vi "Test Z Axis Motor.vi"(6 "Stop Button":bool, 9 "Motor Test Controls":T1, 10 "PWM Duty Cycle":dbl(knob) min=0.0 max=100.0 step=1.0 scale=0.0..100.0) -> ()   [LabVIEW 2013]
doc: "This VI tests the Z-axis functionality. The Z-axis communicates a bit differently than the X and Y axes, thus\nit is given its own test VI."
uses:
  Controls/PWM_test_ctrl_cluster.ctl
  Controls/PWM_data_cluster.ctl
  Controls/table_axis_enum.ctl
  Controls/PWM_state_enum.ctl
  <vilib>/DAQmx/write.llb/DAQmx Write (Digital Bool 1Line 1Point).vi
  <vilib>/DAQmx/miscellaneous.llb/DAQmx Fill In Error Info.vi
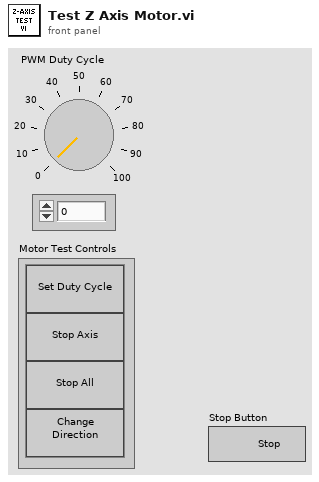
[diagram p1: front panel]
types:
  T1 = typedef "PWM_test_ctrl_cluster.ctl" = cluster{"Set Speed":bool, "Stop Axis":bool, "Stop All":bool, "Change Dir":bool}
  T2 = typedef "PWM_data_cluster.ctl" = cluster{"frequency":dbl, "Duty Cycle (%)":dbl, "Axis Enum":T3, "Function Enum":T4}
  T3 = typedef "table_axis_enum.ctl" = enum16{"X-axis", "Y-axis", "Z-axis", "W-axis"}
  T4 = typedef "PWM_state_enum.ctl" = enum16{"Initialize", "SetAxisSpeed", "StopAxis", "StopAll", "Shutdown"}
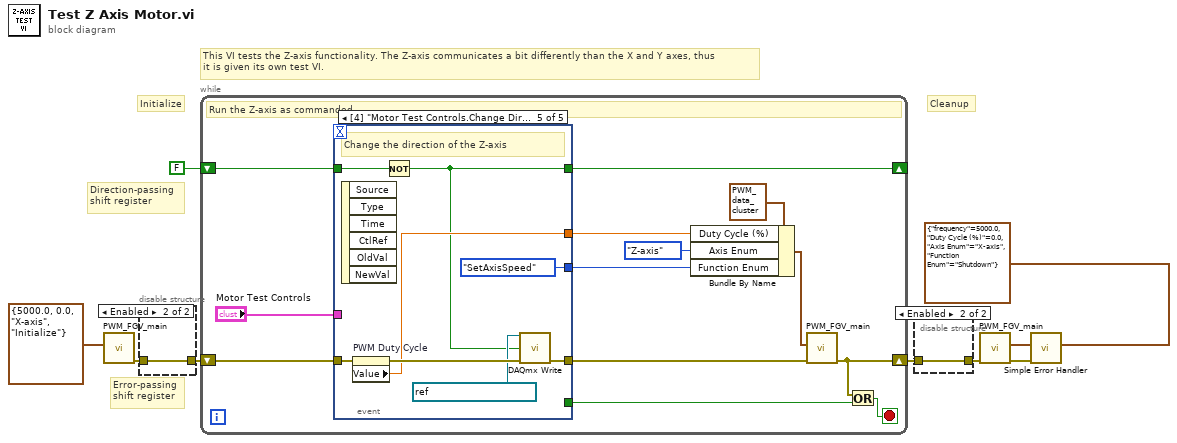
[diagram p0: block diagram]
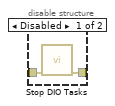
[diagram p2: hidden frame]
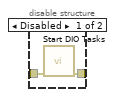
[diagram p3: hidden frame]
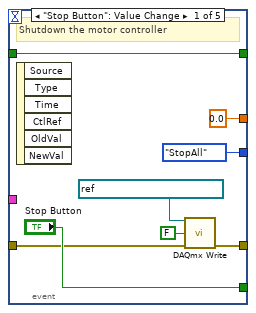
[diagram p4: hidden frame]
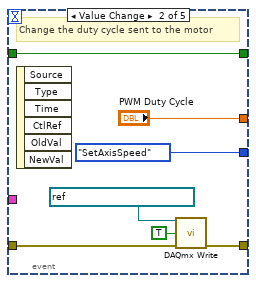
[diagram p5: hidden frame]
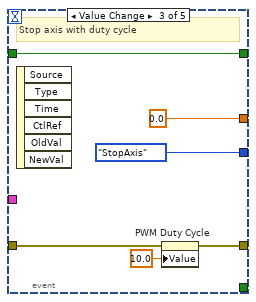
[diagram p6: hidden frame]
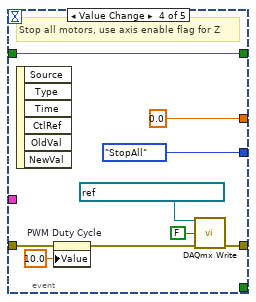
[diagram p7: hidden frame]
diagram:
  # "Direction-passing\nshift register"
  # "Cleanup"
  # "Initialize"
  # "Error-passing\nshift register"
  # "This VI tests the Z-axis functionality. The Z-axis communicates a bit differently than the X and Y axes, thus\nit is given its own test VI."
  n1 = call "PWM_FGV_main.vi"("PWM FGV Data"=T2 {"frequency"=5000.0, "Duty Cycle (%)"=0.0, "Axis Enum"=enum."X-axis", "Function Enum"=enum."Initialize"}) -> ("Error Out"=w7:errorcluster)  [unwired: 10 in]
  n2 = disable-structure shown="Enabled" {
    disable-tunnel: w7 -> [w10 w11]
    disable-tunnel: [w9 w11] -> w6
    frame Disabled {
      n3 = call "Start DIO Tasks.vi"("error in (no error)"=w10) -> ("error out"=w9:errorcluster)  [unwired: 10 in]
    }
    frame Enabled {
    }
  }
  n4 = while {
    shift-right: [w21] -> w5
    shift-left: w6 -> [w24]
    shift-right: [w12] -> _
    shift-left: FALSE -> [w13]
    stop <- w22 stop-if-true
    # "Run the Z-axis as commanded"
    n5 = event shown="[4] \"Motor Test Controls.Change Dir\": Value Change" {
      selector: _ -> [_ _ _ _ _]
      dyn-events: _ -> [_ _ _ _ _]
      timeout: _ -> [_ _ _ _ _]
      tunnel: w24 -> [w28 w36 w43 w52 w61]
      tunnel: "Motor Test Controls" -> [_ _ _ _ _]
      tunnel: [w29 w37 w42 w50 w62] -> w20
      tunnel: ["Stop Button" _ _ _ _] -> w19
      tunnel: [0.0 ("Duty Cycle (%)") "PWM Duty Cycle" 0.0 ("PWM Duty Cycle") 0.0 ("PWM Duty Cycle") w58] -> w16
      tunnel: [PWM_state_enum."StopAll" ("Function Enum") PWM_state_enum."SetAxisSpeed" ("Function Enum") PWM_state_enum."StopAxis" ("Function Enum") PWM_state_enum."StopAll" ("Function Enum") PWM_state_enum."SetAxisSpeed" ("Function Enum")] -> w15
      tunnel: w13 -> [w25 w33 w40 w46 w56]
      tunnel: [w25 w33 w40 w46 w55] -> w12
      event "Stop Button": Value Change {
        # "Shutdown the motor controller"
        n6 = event-data() -> ()  [unwired: 1 in, 6 out]
        n7 = call-poly <vilib>:"DAQmx Write.vi"("task/channels in"=refnum<k21> "ZmotorEnable_S4P0L0", "data"=FALSE, "error in"=w28) -> ("error out"=w29:errorcluster)  [unwired: 10 in, 2 out]
      }
      event Value Change {
        # "Change the duty cycle sent to the motor"
        n8 = event-data() -> ()  [unwired: 1 in, 6 out]
        n9 = call-poly <vilib>:"DAQmx Write.vi"("task/channels in"=refnum<k21> "ZmotorEnable_S4P0L0", "data"=TRUE, "error in"=w36) -> ("error out"=w37:errorcluster)  [unwired: 10 in, 2 out]
      }
      event Value Change {
        # "Stop axis with duty cycle"
        n10 = event-data() -> ()  [unwired: 1 in, 6 out]
        n11 = property on="PWM Duty Cycle" class="Knob (strict)"(error in=w43, "Value"=10.0 ("PWM Duty Cycle")) -> (error out=w42:errorcluster)  [unwired: 1 in, 1 out]
      }
      event Value Change {
        # "Stop all motors, use axis enable flag for Z"
        n12 = event-data() -> ()  [unwired: 1 in, 6 out]
        n13 = property on="PWM Duty Cycle" class="Knob (strict)"(error in=w52, "Value"=10.0 ("PWM Duty Cycle")) -> (error out=w49:errorcluster)  [unwired: 1 in, 1 out]
        n14 = call-poly <vilib>:"DAQmx Write.vi"("task/channels in"=refnum<k21> "ZmotorEnable_S4P0L0", "data"=FALSE, "error in"=w49) -> ("error out"=w50:errorcluster)  [unwired: 10 in, 2 out]
      }
      event Value Change {
        # "Change the direction of the Z-axis"
        n15 = event-data() -> ()  [unwired: 1 in, 6 out]
        n16 = property on="PWM Duty Cycle" class="Knob (strict)"(error in=w61) -> (error out=w60:errorcluster, "Value"=w58:dbl)  [unwired: 1 in, 1 out]
        n17 = Not(x=w56) -> (.not. x?=w55:bool)
        n18 = call-poly <vilib>:"DAQmx Write.vi"("task/channels in"=refnum<k21> "Zdirection_S4P0L1", "data"=w55, "error in"=w60) -> ("error out"=w62:errorcluster)  [unwired: 10 in, 2 out]
      }
    }
    n19 = Bundle By Name(cluster=T2 {"frequency"=5000.0, "Duty Cycle (%)"=0.0, "Axis Enum"=enum."X-axis", "Function Enum"=enum."Shutdown"} ("PWM FGV Data"), "Duty Cycle (%)"=w16, "Axis Enum"=table_axis_enum."Z-axis", "Function Enum"=w15) -> (w17:T2)
    n20 = call "PWM_FGV_main.vi"("Error In"=w20, "PWM FGV Data"=w17) -> ("Error Out"=w21:errorcluster)  [unwired: 9 in]
    n21 = Or(x=w21, y=w19) -> (x .or. y?=w22:bool)
  }
  n22 = disable-structure shown="Enabled" {
    disable-tunnel: w5 -> [w64 w65]
    disable-tunnel: [w63 w65] -> w4
    frame Disabled {
      n23 = call "Stop DIO Tasks.vi"("Error In"=w64) -> ("error out"=w63:errorcluster)  [unwired: 10 in]
    }
    frame Enabled {
    }
  }
  n24 = call "PWM_FGV_main.vi"("Error In"=w4, "PWM FGV Data"=T2 {"frequency"=5000.0, "Duty Cycle (%)"=0.0, "Axis Enum"=enum."X-axis", "Function Enum"=enum."Shutdown"}) -> ("Error Out"=w2:errorcluster)  [unwired: 9 in]
  n25 = call <vilib>:"Simple Error Handler.vi"("error in (no error)"=w2) -> ()  [unwired: 4 in, 5 out]
